vi "Peak.vi"(0 "VisaCluster":T1, 7 "Peak":bool, 11 "error in (no error)":errorcluster) -> (4 "VisaCluster":T1, 6 "Peak":bool, 8 "Answer":string, 10 "Display":string, 15 "error out":errorcluster)   [LabVIEW 2014, in "FH 55.lvlib"]
doc: "This VI sets the PEAK ON or OFF.\n\nDurch diese VI kann die Peak-Funktion an- und ausgeschaltet werden. Die Funktion dient zur Messung von Impulsfeldern oder des Spitzenwerts von Wechselfeldern."
uses:
  FH 55.lvlib
  TypeDef/VisaCluster.ctl
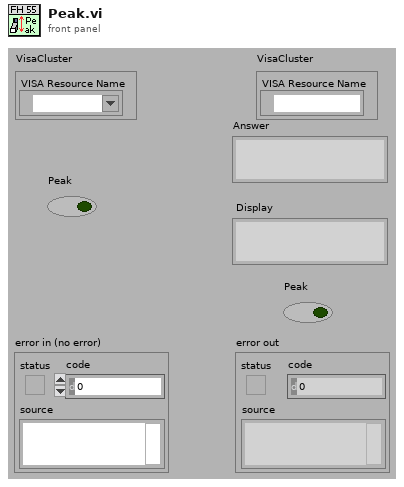
[diagram p1: front panel]
types:
  T1 = typedef "FH 55.lvlib/VisaCluster.ctl" = cluster{"VISA Resource Name":refnum<visa-resource-name>}
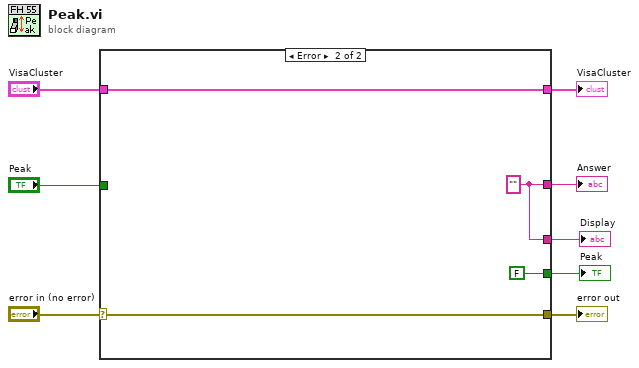
[diagram p0: block diagram]
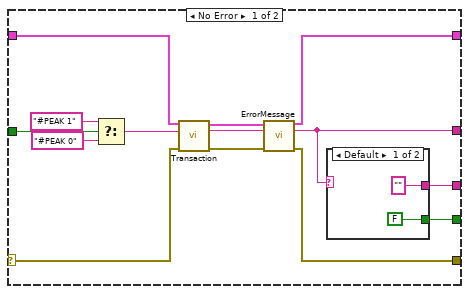
[diagram p2: hidden frame]
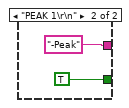
[diagram p3: hidden frame]
diagram:
  n1 = case shown="Error" "error in (no error)" {
    selector: "error in (no error)" -> [w15 w29]
    tunnel: "VisaCluster" -> [w17 w30]
    tunnel: "Peak" -> [w22 _]
    tunnel: [w19 w30] -> w4
    tunnel: [w18 w29] -> w6
    tunnel: [w11 w28] -> w5
    tunnel: [w10 w28] -> w2
    tunnel: [w9 FALSE] -> w1
    frame No Error {
      n2 = Select(t="#PEAK 1", s=w22, f="#PEAK 0") -> (s? t:f=w16:string)
      n3 = call "Transaction.vi"("VisaCluster"=w17, "Command"=w16, "error in (no error)"=w15) -> ("VisaCluster"=w12:T1, "Answer"=w13:string, "error out"=w14:errorcluster)  [unwired: 9 in, 1 out]
      n4 = call "ErrorMessage.vi"("VisaCluster"=w12, "Message In"=w13, "error in (no error)"=w14) -> ("VisaCluster"=w19:T1, "Message Out"=w11:string, "error out"=w18:errorcluster)  [unwired: 10 in]
      n5 = case shown="Default" w11 {
        tunnel: ["" "-Peak"] -> w10
        tunnel: [FALSE TRUE] -> w9
        frame Default {
        }
        frame "PEAK 1\r\n" {
        }
      }
    }
    frame Error {
      w28 = ""
    }
  }
  "error out" <- w6
  "Answer" <- w5
  "VisaCluster" <- w4
  "Display" <- w2
  "Peak" <- w1
